vi "Neighbors.vi"(11 "Square in":refnum<class "Square.lvclass">) -> (2 "Neighbors":i32[](array[numeric]))   [LabVIEW 2020, in "SquareBattle.lvlib" / "Square.lvclass"]
doc: "Returns the team index of all neighboring positions for the square. The neighbors start in the NW and continue clockwise and the index also matches the value of the Direction.ctl values."
uses:
  Square.lvclass
  Square.lvclass/Square.ctl
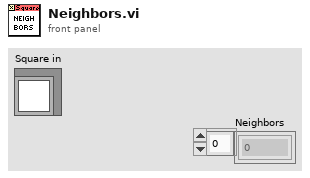
[diagram p1: front panel]
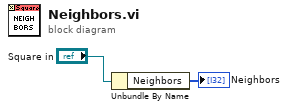
[diagram p0: block diagram]
diagram:
  n1 = Unbundle By Name("Square in") -> ("Neighbors"=→"Neighbors":i32[])
